vi "Unicode Tree File Browser Example.vi"() -> ()   [LabVIEW 2020]
doc: "This VI demonstrates a tree based file browser with unicode support."
uses:
  Types/UTF-8 String/UTF-8 String.lvclass
  Types/UTF-8 String/UTF-8 String.lvclass/UTF-8 String.ctl
  Types/UTF-8 Path/UTF-8 Path.lvclass/UTF-8 Path.ctl
  Dialog & User Interface/Polymorphic VIs/Write Control Text/Write String Value (UTF-8 String).vi
  aeeff775-071d-483d-8d41-183d596e9df0.vi
  c6942421-cd3a-4fd7-ba65-2311fd5167b5.vi
  Dialog & User Interface/Polymorphic VIs/Write Control Text/Write Listbox Items (UTF-8 String).vi
  Dialog & User Interface/Polymorphic VIs/Write Control Text/Write String Value (UTF-8 String).vi/5206cb6b-04fb-41f5-a37e-29c14f142303.vi
  Private/Conversion/Text as Encoded Path.vi
  Private/Conversion/Polymorphic VIs/Text as Encoded Path (UTF-8 String).vi
  Types/UTF-8 Path/Write Encoded UTF-8 Path.vi
  Private/Conversion/Path as UTF-8 Path.vi
  Private/Conversion/Polymorphic VIs/Path as UTF-8 Path (UTF-8 Path).vi
  c6942421-cd3a-4fd7-ba65-2311fd5167b5.vi/5269e09c-4216-478e-8686-9fb7d38e224a.vi
  c6942421-cd3a-4fd7-ba65-2311fd5167b5.vi/d1f4a45d-6f02-44dd-a40b-2b28d80e6519.vi
  Private/Conversion/String as Encoded String.vi
  Private/Conversion/Polymorphic VIs/String as Encoded String (UTF-8 String).vi
  Private/Library/gu_list_folder.vi
  c6942421-cd3a-4fd7-ba65-2311fd5167b5.vi/8eb4f0ed-0012-4550-978e-be3f7301df70.vi
  c6942421-cd3a-4fd7-ba65-2311fd5167b5.vi/f7e6584c-01ed-423f-9bcd-660954191d0d.vi
  Dialog & User Interface/Polymorphic VIs/Write Control Text/Write Listbox Items (UTF-8 String).vi/5206cb6b-04fb-41f5-a37e-29c14f142303.vi
  Private/Conversion/Text as Encoded String.vi
  Private/Conversion/Polymorphic VIs/Text as Encoded String (UTF-8 String).vi
  Private/Conversion/Encoded UTF-8 String to Encoded UTF-16LE String.vi
  Types/UTF-8 String/Read Encoded UTF-8 String.vi
  c6942421-cd3a-4fd7-ba65-2311fd5167b5.vi/5269e09c-4216-478e-8686-9fb7d38e224a.vi/c24c063b-f849-48a1-b323-238a063d7118.vi
  c6942421-cd3a-4fd7-ba65-2311fd5167b5.vi/5269e09c-4216-478e-8686-9fb7d38e224a.vi/a2fd6c11-d594-45c9-8624-1f0a1df69df3.vi
  c6942421-cd3a-4fd7-ba65-2311fd5167b5.vi/5269e09c-4216-478e-8686-9fb7d38e224a.vi/1fd3173e-d32e-42cb-8f0d-819132eb8e27.vi
  c6942421-cd3a-4fd7-ba65-2311fd5167b5.vi/5269e09c-4216-478e-8686-9fb7d38e224a.vi/bb7c39fc-ad8e-447d-bc50-468674bfb562.vi
  Private/Conversion/Polymorphic VIs/Text as Encoded String (UTF-8 Path).vi
  Private/Library/Result To Error.vi
  c6942421-cd3a-4fd7-ba65-2311fd5167b5.vi/8eb4f0ed-0012-4550-978e-be3f7301df70.vi/3a31b270-3bb6-4c58-a256-c5fcc2c98f09.vi
  c6942421-cd3a-4fd7-ba65-2311fd5167b5.vi/8eb4f0ed-0012-4550-978e-be3f7301df70.vi/0ec5df2d-ef9b-4f84-a6a8-ffcedd45c4dc.vi
  Private/Conversion/Text as String.vi
  Private/Conversion/Polymorphic VIs/Text as String (UTF-8 Path).vi
  Private/Conversion/Path as Encoded Path.vi
  Private/Conversion/Polymorphic VIs/Path as Encoded Path (UTF-8 Path).vi
  Private/Library/gu_string_subset.vi
  Private/Library/gu_to_lower_case.vi
  Private/Library/gu_search_split_string.vi
  Private/Conversion/Polymorphic VIs/String as Encoded String (LabVIEW String).vi
  Types/UTF-8 Path/Read Encoded UTF-8 Path.vi
  Private/Conversion/Polymorphic VIs/Text as Encoded String (LabVIEW String).vi
  Private/Memory/Copy String.vi
  Private/Conversion/Text to UTF-8.vi
  Private/Conversion/Polymorphic VIs/Text to UTF-8 (LabVIEW String).vi
  Private/Memory/Copy String.vi/4d47babd-4a2d-4eb7-b91b-7e707d692665.vi
  Private/Library/gu_free.vi
  Private/User Interface/Write String.vi
  <vilib>/Utility/error.llb/Error Cluster From Error Code.vi
  Private/Memory/Copy String Array.vi
  File IO/Path to Short Name (Unicode).vi
  Private/User Interface/Write Listbox Data.vi
  Types/UTF-8 Path/UTF-8 Path.lvclass
  Tree Browser/Tree Browser.lvlib
  G-Unicode.lvlib
panel:
  in  "Path":string
  in  "File List":i32(listbox)=-1
  in  "Directory Tree":string(tree)
  # "Instructions:\n1. Run the VI.\n2. Browse the directory tree on the left. Note it displays any unicode folders.\n3. Select a folder in the tree to see its contents on the right. Note it displays any unicode files.\n4. Collapse and expand a tree item to refresh its contents."
  # "G"
  # "-Unicode"
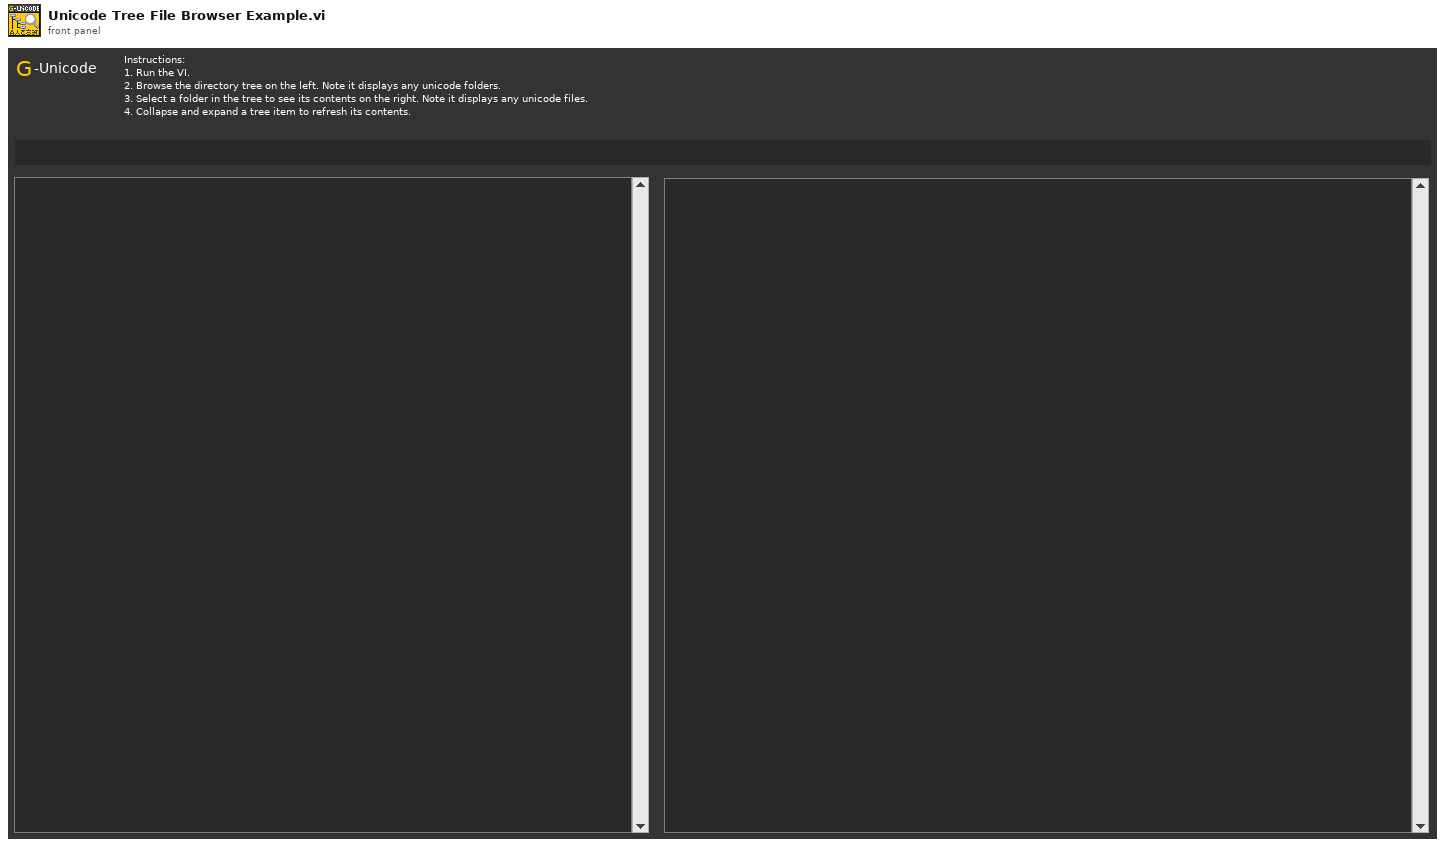
[diagram p1: front panel]
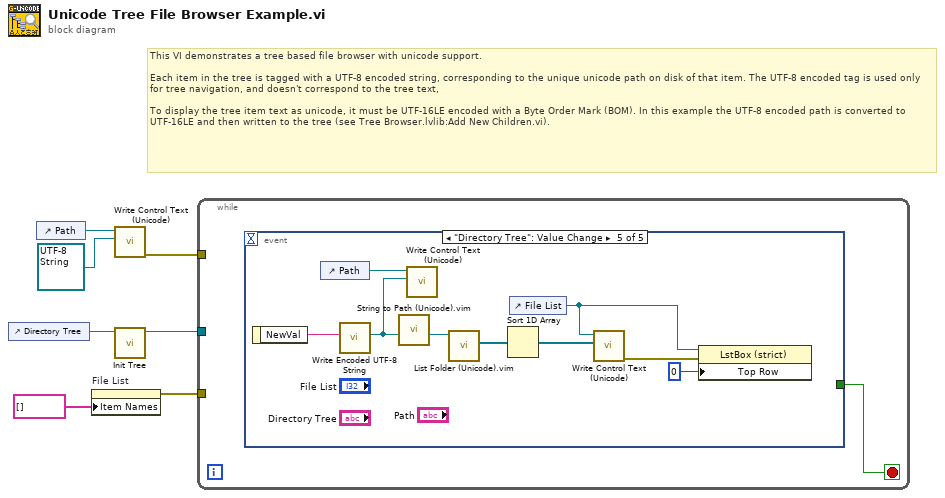
[diagram p0: block diagram]
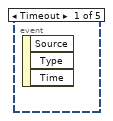
[diagram p2: hidden frame]
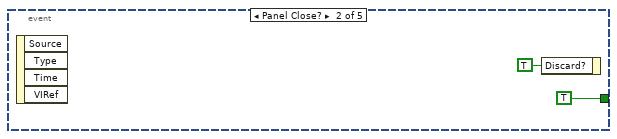
[diagram p3: hidden frame]
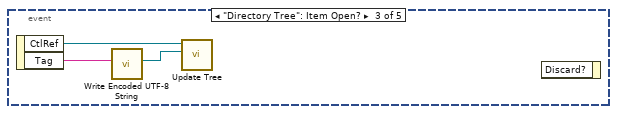
[diagram p4: hidden frame]
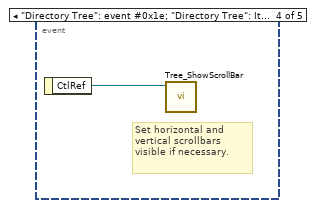
[diagram p5: hidden frame]
diagram:
  # "This VI demonstrates a tree based file browser with unicode support.\n\nEach item in the tree is tagged with a UTF-8 encoded string, corresponding to the unique unicode path on disk of that item. The UTF-8 encoded tag is used only for tree navigation, and doesn't correspond to the tree text,\n\nTo display the tree item text as unicode, it must be UTF-16LE encoded with a Byte Order Mark (BOM). In this example the UTF-8 encoded path is converted to UTF-16LE and then written to the tree (see Tree Browser.lvlib:Add New Children.vi)."
  n1 = control-ref of="Directory Tree"() -> (w6:refnum<vi>)
  n2 = control-ref of="Path"() -> (w3:refnum<vi>)
  n3 = property on="File List" class="LstBox (strict)"("Item Names"=string[] []) -> (error out=w5:errorcluster)  [unwired: 2 in, 1 out]
  n4 = call-poly "Write Control Text (Unicode).vi"("Value"=refnum<class "UTF-8 String.lvclass"> refnum ("G-Unicode.lvlib:UTF-8 String.lvclass"), "Control Ref"=w3) -> ("error out"=w2:errorcluster)  [unwired: 9 in]
  n5 = call "Init Tree.vi"("Tree In"=w6) -> ("Tree Out"=w4:refnum<vi>)  [unwired: 10 in]
  n6 = while {
    tunnel: w5 -> [_]
    tunnel: w4 -> [_]
    tunnel: w2 -> [_]
    stop <- w8 stop-if-true
    n7 = event shown="[4] \"Directory Tree\": Value Change" {
      selector: _ -> [_ _ _ _ _]
      dyn-events: _ -> [_ _ _ _ _]
      timeout: _ -> [_ _ _ _ _]
      tunnel: [_ TRUE _ _ _] -> w8
      event Timeout {
        n8 = event-data() -> ()  [unwired: 1 in, 3 out]
      }
      event Panel Close? {
        n9 = event-data() -> ()  [unwired: 1 in, 4 out]
        n10 = event-data("Discard?"=TRUE) -> ()  [unwired: 1 in, 1 out]
      }
      event "Directory Tree": Item Open? {
        n11 = event-data() -> ("CtlRef"=w13:refnum<vi>, "Tag"=w12:string)  [unwired: 1 in]
        n12 = call "Write Encoded UTF-8 String.vi"("Encoded UTF-8 String"=w12) -> ("UTF-8 String"=w11:refnum<class "UTF-8 String.lvclass">)  [unwired: 10 in]
        n13 = call "Update Tree.vi"("Parent Tag"=w11, "Tree In"=w13) -> ()  [unwired: 9 in, 1 out]
        n14 = event-data() -> ()  [unwired: 2 in, 1 out]
      }
      event "Directory Tree": event #0x1e; "Directory Tree": Item Close {
        # "Set horizontal and vertical scrollbars visible if necessary."
        n15 = event-data() -> ("CtlRef"=w14:refnum<vi>)  [unwired: 1 in]
        n16 = call <vilib>:"Tree_ShowScrollBar.vi"("Tree"=w14) -> ()  [unwired: 10 in, 1 out]
      }
      event "Directory Tree": Value Change {
        n17 = event-data() -> ("NewVal"=w21:string)  [unwired: 1 in]
        n18 = control-ref of="Path"() -> (w18:refnum<vi>)
        n19 = call "Write Encoded UTF-8 String.vi"("Encoded UTF-8 String"=w21) -> ("UTF-8 String"=w17:refnum<class "UTF-8 String.lvclass">)  [unwired: 10 in]
        n20 = call "String to Path (Unicode).vim"("String"=w17) -> ("Path"=w22:refnum<class "UTF-8 Path.lvclass">)  [unwired: 9 in, 1 out]
        n21 = call-poly "Write Control Text (Unicode).vi"("Value"=w17, "Control Ref"=w18) -> ()  [unwired: 9 in, 1 out]
        n22 = call "List Folder (Unicode).vim"("Path"=w22) -> ("Filenames"=w23:refnum<class "UTF-8 String.lvclass">[])  [unwired: 7 in, 3 out]
        n23 = Sort 1D Array(array=w23) -> (sorted array=w20:refnum<class "UTF-8 String.lvclass">[])
        n24 = control-ref of="File List"() -> (w15:refnum<vi>)
        n25 = call-poly "Write Control Text (Unicode).vi"("Value"=w20, "Control Ref"=w15) -> ("error out"=w16:errorcluster)  [unwired: 9 in]
        n26 = property class="LstBox (strict)"(reference=w15, error in=w16, "Top Row"=0) -> ()  [unwired: 2 out]
      }
    }
  }
